vi "ex7-12.vi"() -> ()   [LabVIEW 2013]
panel:
  out "initialized array":dbl[](array[numeric])
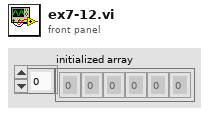
[diagram p1: front panel]
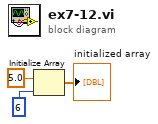
[diagram p0: block diagram]
diagram:
  n1 = Initialize Array(5.0 ("element"), 6 ("dimension size")) -> (→"initialized array":dbl[])
